vi "TestMain UI.vi"() -> ()   [LabVIEW 2016]
panel:
  in  "Numeric":dbl
  in  "stop":bool
  in  "AdujstSplit 4":bool
  in  "Clear":bool
  in  "Save":bool
  in  "DeletePage":bool
  in  "Page":u16(ring) items=["Page0"]
  in  "AddPage":bool
  in  "Stop":bool
  in  "Run":bool
  in  "Pause":bool
  in  "DeletePanel":bool
  in  "AddPanel":bool
  in  "AdujstSplit 10":bool
  in  "AdujstSplit 9":bool
  in  "AdujstSplit 8":bool
  in  "AdujstSplit 7":bool
  in  "AdujstSplit 5":bool
  in  "AdujstSplit 3":bool
  in  "Tree":string(tree)
  out "Graph":waveform(dbl)(graph) caption="虚拟通道波形"
  in  "Multicolumn Listbox":i32(listbox)
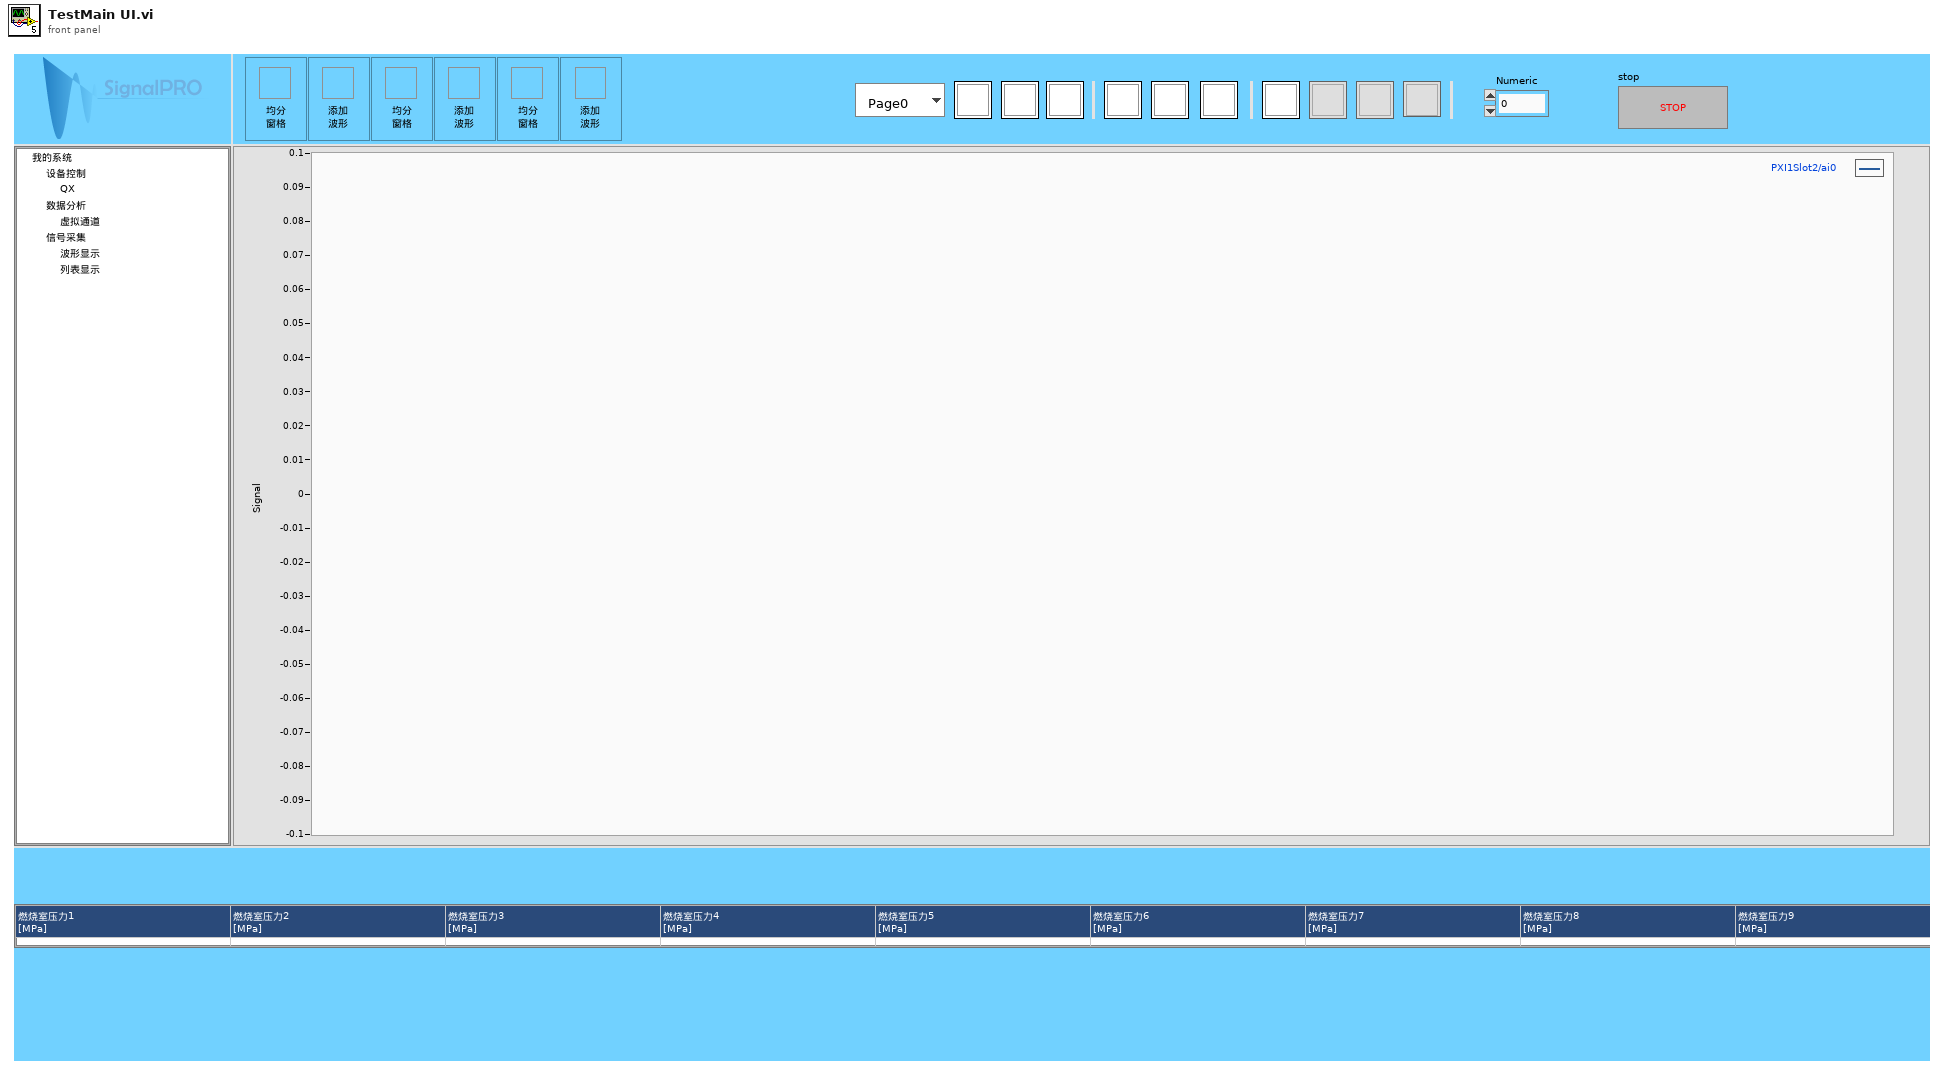
[diagram p1: front panel]
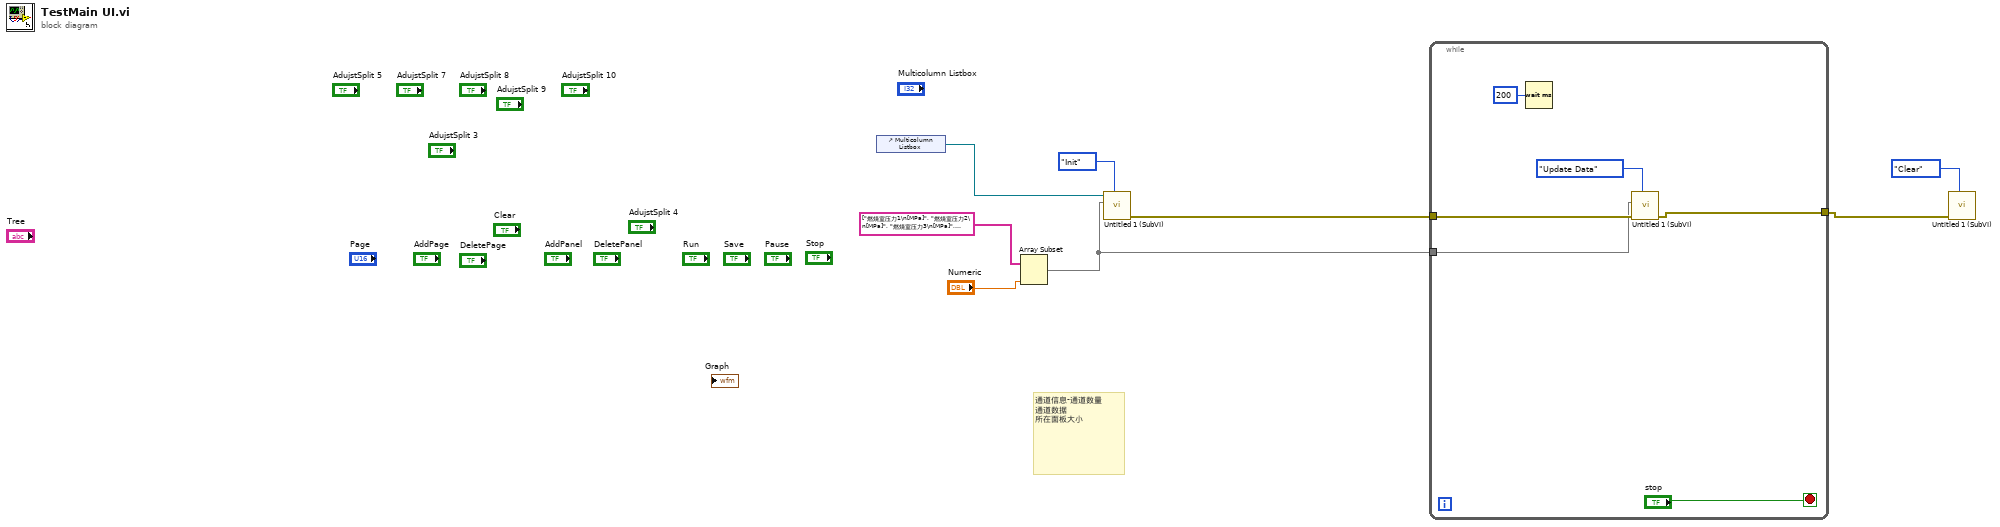
[diagram p0: block diagram]
diagram:
  # "通道信息-通道数量\n通道数据\n所在面板大小"
  n1 = control-ref of="Multicolumn Listbox"() -> (w1:refnum<vi>)
  n2 = Array Subset(array=string[] ["燃烧室压力1\n[MPa]", "燃烧室压力2\n[MPa]", "燃烧室压力3\n[MPa]", "燃烧室压力4\n[MPa]", "燃烧室压力5\n[MPa]", "燃烧室压力6\n[MPa]", "燃烧室压力7\n[MPa]", "燃烧室压力8\n[MPa]", "燃烧室压力9\n[MPa]", "燃烧室压力10\n[MPa]", "燃烧室压力11\n[MPa]", "燃烧室压力12\n[MPa]", "燃烧室压力13\n[MPa]", "燃烧室压力14\n[MPa]", "燃烧室压力15\n[MPa]", "燃烧室压力16\n[MPa]"] ("Channels info"), length="Numeric") -> (w7:string[])  [unwired: 1 in]
  n3 = call "Untitled 1 (SubVI).vi"("Comm"=enum16{"Init", "Clear", "Update Data"}."Init", "Channels info"=w7, "ML Ref"=w1) -> ("error out"=w6:errorcluster)  [unwired: 8 in]
  n4 = while {
    tunnel: w6 -> [w13]
    tunnel: w7 -> [w12]
    tunnel: [w10] -> w4
    stop <- "stop" stop-if-true
    n5 = Wait (ms)(milliseconds to wait=u32 200) -> ()  [unwired: 1 out]
    n6 = call "Untitled 1 (SubVI).vi"("Comm"=enum16{"Init", "Clear", "Update Data"}."Update Data", "error in (no error)"=w13, "Channels info"=w12) -> ("error out"=w10:errorcluster)  [unwired: 8 in]
  }
  n7 = call "Untitled 1 (SubVI).vi"("Comm"=enum16{"Init", "Clear", "Update Data"}."Clear", "error in (no error)"=w4) -> ()  [unwired: 9 in, 1 out]
